vi "Write Coordinates.vi"(10 "Coordinates":T1, 11 "Game Componants in":refnum<class "Game Componants.lvclass">) -> (3 "Game Componants out":refnum<class "Game Componants.lvclass">)   [LabVIEW 2021, in "Game Componants.lvclass"]
doc: "MIT Licence\nCopyright (c) 2024 David Grollier"
uses:
  Game Componants.lvclass
  Type Def/Coordinates.ctl
  Game Componants.lvclass/Game Componants.ctl
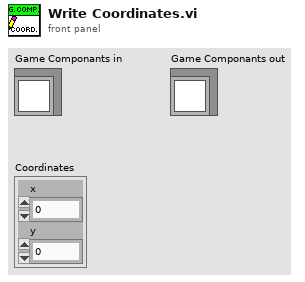
[diagram p1: front panel]
types:
  T1 = typedef "Coordinates.ctl" = cluster{"x":dbl, "y":dbl}
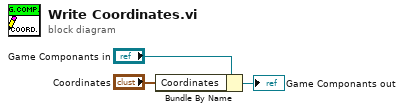
[diagram p0: block diagram]
diagram:
  n1 = Bundle By Name(cluster="Game Componants in", "Coordinates"="Coordinates") -> (→"Game Componants out":refnum<class "Game Componants.lvclass">)
